vi "Constant - Blank Module Data.vi"() -> (0 "Blank Module Data":T1)   [LabVIEW 2023, in "Error Manager.lvlib"]
doc: "Blank VI with error handling."
uses:
  Error Manager.lvlib
  Module Data (cluster).ctl
  Handled Error (cluster).ctl
  Read-Unread Status (enum).ctl
  Display Order (enum).ctl
  Error in current one-second interval (cluster).ctl
panel:
  # "Input\nInputs to the VI"
  # "Development\nControls or indicators that are useful for development or testing, but which are not outputs of the VI."
  # "Output\nOutputs of the VI"
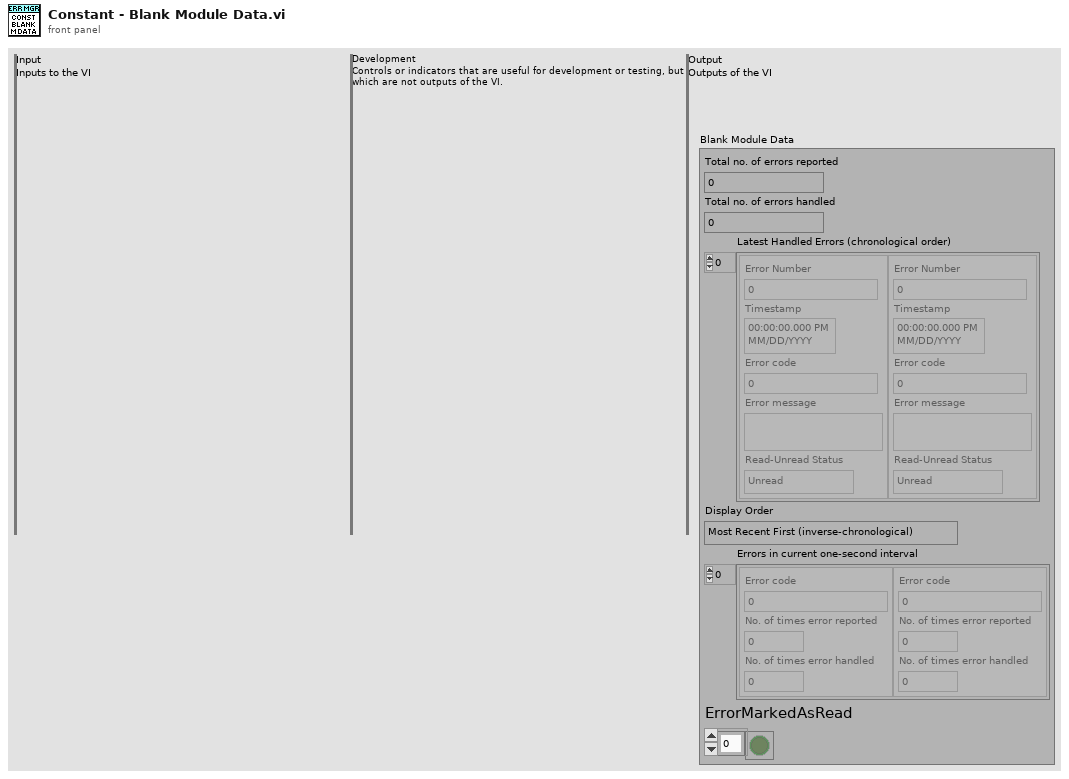
[diagram p1: front panel]
types:
  T1 = typedef "Error Manager.lvlib/Module Data (cluster).ctl" = cluster{"Total no. of errors reported":i32, "Total no. of errors handled":i32, "Latest Handled Errors (chronological order)":T2[], "Display Order":T4, "Errors in current one-second interval":T5[], "ErrorMarkedAsRead":bool[]}
  T2 = typedef "Error Manager.lvlib/Handled Error (cluster).ctl" = cluster{"Error Number":i32, "Timestamp":timestamp, "Error code":i32, "Error message":string, "Read-Unread Status":T3}
  T3 = typedef "Error Manager.lvlib/Read-Unread Status (enum).ctl" = enum16{"Unread", "Read"}
  T4 = typedef "Error Manager.lvlib/Display Order (enum).ctl" = enum16{"Most Recent First (inverse-chronological)", "Oldest First (chronological)"}
  T5 = typedef "Error Manager.lvlib/Error in current one-second interval (cluster).ctl" = cluster{"Error code":i32, "No. of times error reported":u32, "No. of times error handled":u32}
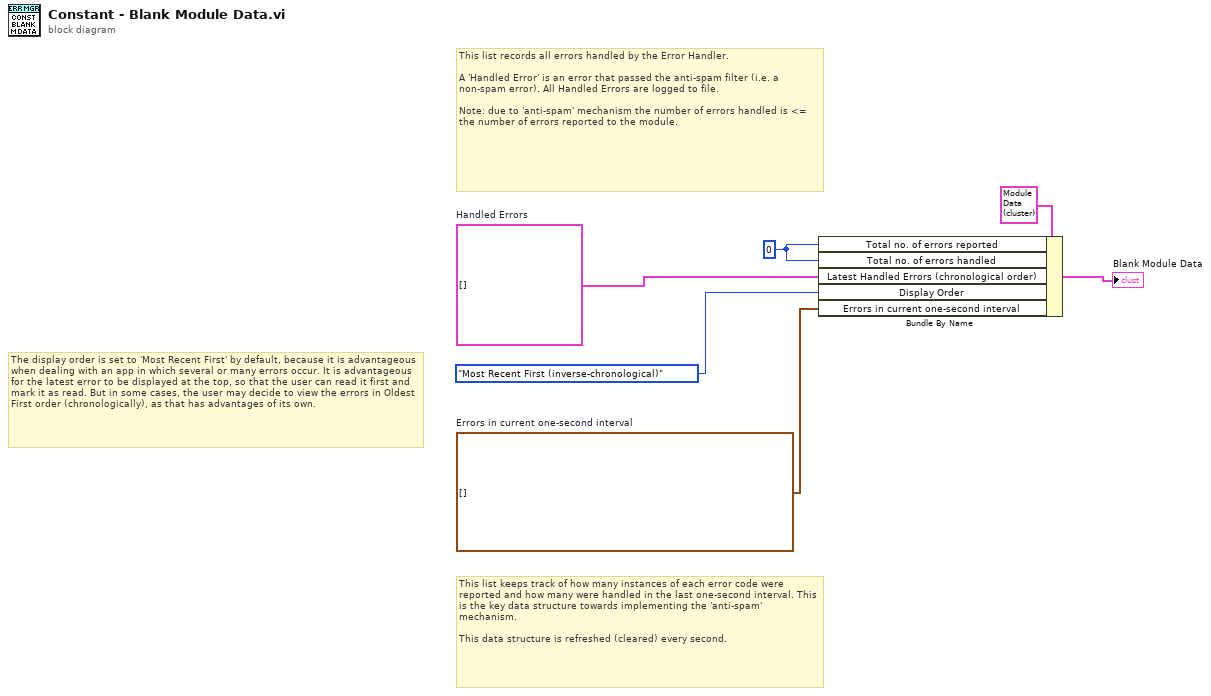
[diagram p0: block diagram]
diagram:
  w1 = 0 ("Total no. of errors handled so far")
  w4 = T5[] []  # Errors in current one-second interval
  w6 = T2[] []  # Handled Errors
  # "This list keeps track of how many instances of each error code were reported and how many were handled in the last one-second interval. This is the key data structure towards implementing the 'anti-spam' mechanism.\n\nThis data structure is refreshed (cleared) every second."
  # "This list records all errors handled by the Error Handler. \n\nA 'Handled Error' is an error that passed the anti-spam filter (i.e. a non-spam error). All Handled Errors are logged to file.\n\nNote: due to 'anti-spam' mechanism the number of errors handled is <= the number of errors reported to the module."
  # "The display order is set to 'Most Recent First' by default, because it is advantageous when dealing with an app in which several or many errors occur. It is advantageous for the latest error to be displayed at the top, so that the user can read it first and mark it as read. But in some cases, the user may decide to view the errors in Oldest First order (chronologically), as that has advantages of its own."
  n1 = Bundle By Name(cluster=T1 {"Total no. of errors reported"=0, "Total no. of errors handled"=0, "Latest Handled Errors (chronological order)"=[], "Display Order"=enum."Most Recent First (inverse-chronological)", "Errors in current one-second interval"=[], "ErrorMarkedAsRead"=[]} ("Module Data"), "Total no. of errors reported"=w1, "Total no. of errors handled"=w1, "Latest Handled Errors (chronological order)"=w6, "Display Order"=Display_Order_(enum)."Most Recent First (inverse-chronological)", "Errors in current one-second interval"=w4) -> (→"Blank Module Data":T1)
